vi "Motion UI.vi"() -> ()   [LabVIEW 2010]
uses:
  Motion_Gantry Position.ctl
  Motion_Coils Typedef.ctl
  Motion_Registers Typedef.ctl
  <vilib>/NI Modbus.llb/MB Ethernet Master Query Write Multiple Registers (poly).vi
panel:
  in  "Write Home data\n(All Axis)":bool
  in  "X Home Data":T1={"Approach Velocity (In/Sec)"=1.0, "Creep Velocity (In/Sec)"=0.5, "Offset (In)"=-0.0625, "OffsetVelocity (In/Sec)"=0.5, "AccDec\n(In/Sec/Sec)"=1.0, "Position (In)"=22.525} {"Position (In)" format="%.3f"; "AccDec\n(In/Sec/Sec)" min=0.01 max=20.0 format="%.2f"; "OffsetVelocity (In/Sec)" min=0.01 max=2.0 format="%.2f"; "Offset (In)" min=-1.0 max=1.0 format="%.3f"; "Creep Velocity (In/Sec)" min=0.5 max=1.0 format="%.2f"; "Approach Velocity (In/Sec)" min=0.01 max=2.0 format="%.2f"}
  in  "Y Home Data":T2={"Approach Velocity\n(In/Sec)"=1.0, "Creep Velocity\n(In/Sec)"=0.5, "Offset (In)"=-0.0625, "OffsetVelocity\n(In/Sec)"=0.5, "AccDec\n(In/Sec/Sec)"=1.0, "Position (In)"=5.9} {"Position (In)" format="%.3f"; "AccDec\n(In/Sec/Sec)" min=0.01 max=20.0 format="%.2f"; "OffsetVelocity\n(In/Sec)" min=0.01 max=2.0 format="%.2f"; "Offset (In)" min=-1.0 max=1.0 format="%.3f"; "Creep Velocity\n(In/Sec)" min=0.5 max=1.0 format="%.2f"; "Approach Velocity\n(In/Sec)" min=0.01 max=2.0 format="%.2f"}
  in  "Z Home Data":T2={"Approach Velocity\n(In/Sec)"=1.0, "Creep Velocity\n(In/Sec)"=0.5, "Offset (In)"=-0.0625, "OffsetVelocity\n(In/Sec)"=0.5, "AccDec\n(In/Sec/Sec)"=1.0, "Position (In)"=5.75} {"Position (In)" format="%.3f"; "AccDec\n(In/Sec/Sec)" min=0.01 max=20.0 format="%.2f"; "OffsetVelocity\n(In/Sec)" min=0.01 max=2.0 format="%.2f"; "Offset (In)" min=-1.0 format="%.3f"; "Creep Velocity\n(In/Sec)" min=0.5 max=1.0 format="%.2f"; "Approach Velocity\n(In/Sec)" min=0.01 max=2.0 format="%.2f"}
  in  "Loader Home Data":T2={"Approach Velocity\n(In/Sec)"=1.0, "Creep Velocity\n(In/Sec)"=0.5, "Offset (In)"=0.0625, "OffsetVelocity\n(In/Sec)"=0.5, "AccDec\n(In/Sec/Sec)"=1.0, "Position (In)"=0.0} {"Position (In)" min=0.0 max=1.0 format="%.3f"; "AccDec\n(In/Sec/Sec)" min=0.01 max=20.0 format="%.2f"; "OffsetVelocity\n(In/Sec)" min=0.01 max=2.0 format="%.2f"; "Offset (In)" min=-1.0 max=1.0 format="%.3f"; "Creep Velocity\n(In/Sec)" min=0.5 max=1.0 format="%.2f"; "Approach Velocity\n(In/Sec)" min=0.01 max=2.0 format="%.2f"}
  out "Errors":cluster{"Error ID":u16, "Error String":string}[](array[cluster])
  in  "General Alarm Clear":bool
  out "Loader Discretes":T3
  out "Gantry Discretes":T4
  out "Gantry Position":T5
  out "error out":errorcluster
  in  "stop":bool
  in  "address:port":string="192.168.0.3:502"
  in  "Gantry Move Data":T6={"Gantry Accel/Decel"=5.0, "Gantry Velocity"=5.0, "X-Position"=0.3, "Y-Position"=0.0, "Z-Position"=-0.5} {"Z-Position" format="%_7g"; "Y-Position" format="%_7g"; "X-Position" format="%_7g"; "Gantry Velocity" format="%_7g"; "Gantry Accel/Decel" format="%_7g"}
  out "Loader Actual Position":dbl format="%.3f"
  in  "Loader Stop":bool
  in  "Loader Goto Load":bool
  in  "Loader Goto Connect":bool
  in  "Loader Enable":bool
  in  "Loader Home":bool
  in  "Gantry Goto":bool
  in  "Gantry Home":bool
  in  "Gantry Enable":bool
  # "Loader Control"
  # "Gantry Control"
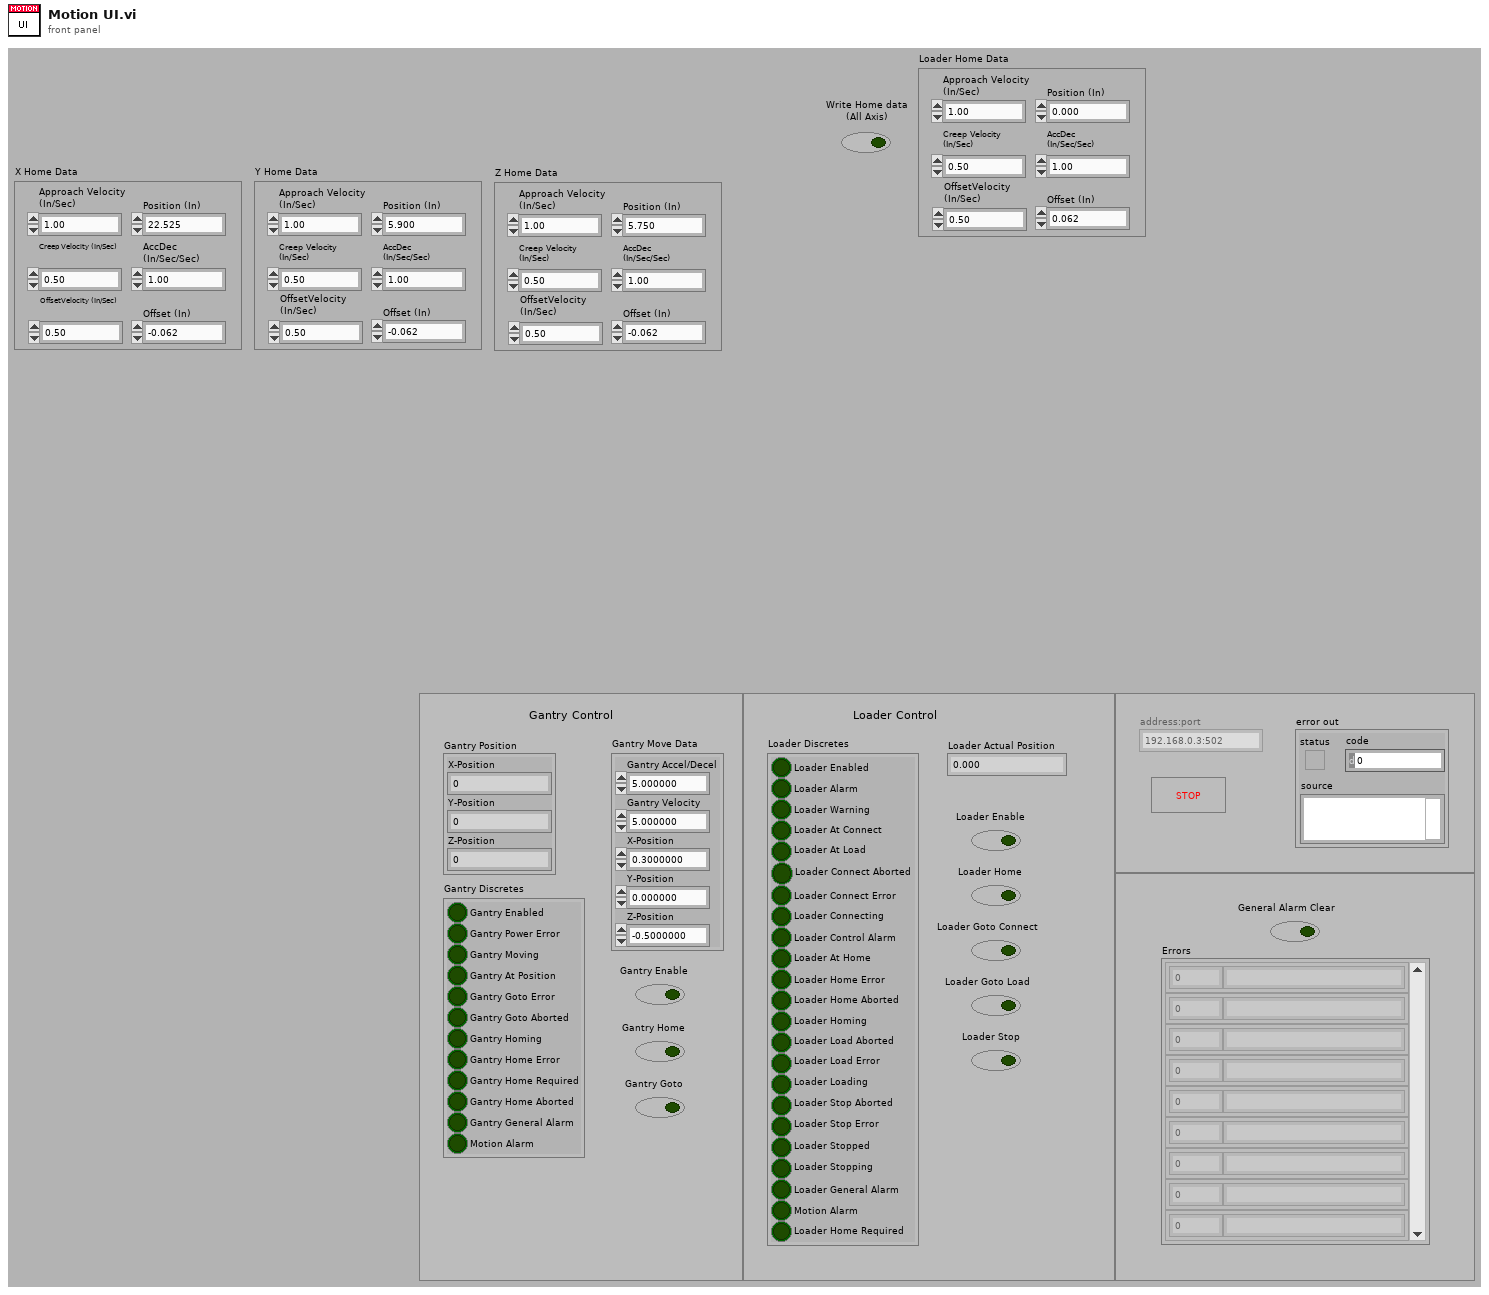
[diagram p1: front panel]
types:
  T1 = cluster{"Approach Velocity (In/Sec)":dbl, "Creep Velocity (In/Sec)":dbl, "Offset (In)":dbl, "OffsetVelocity (In/Sec)":dbl, "AccDec\n(In/Sec/Sec)":dbl, "Position (In)":dbl}
  T2 = cluster{"Approach Velocity\n(In/Sec)":dbl, "Creep Velocity\n(In/Sec)":dbl, "Offset (In)":dbl, "OffsetVelocity\n(In/Sec)":dbl, "AccDec\n(In/Sec/Sec)":dbl, "Position (In)":dbl}
  T3 = cluster{"Loader Enabled":bool, "Loader Alarm ":bool, "Loader Warning":bool, "Loader At Connect":bool, "Loader At Load":bool, "Loader Connect Aborted":bool, "Loader Connect Error":bool, "Loader Connecting":bool, "Loader Control Alarm":bool, "Loader At Home":bool, "Loader Home Error":bool, "Loader Home Aborted":bool, "Loader Homing":bool, "Loader Load Aborted":bool, "Loader Load Error":bool, "Loader Loading":bool, "Loader Stop Aborted":bool, "Loader Stop Error":bool, "Loader Stopped":bool, "Loader Stopping":bool, "Loader General Alarm":bool, "Motion Alarm":bool, "Loader Home Required":bool}
  T4 = cluster{"Gantry Enabled":bool, "Gantry Power Error":bool, "Gantry Moving":bool, "Gantry At Position":bool, "Gantry Goto Error":bool, "Gantry Goto Aborted":bool, "Gantry Homing":bool, "Gantry Home Error":bool, "Gantry Home Required":bool, "Gantry Home Aborted":bool, "Gantry General Alarm":bool, "Motion Alarm":bool}
  T5 = cluster{"X-Position":dbl, "Y-Position":dbl, "Z-Position":dbl}
  T6 = typedef "Motion_Gantry Position.ctl" = cluster{"Gantry Accel/Decel":dbl, "Gantry Velocity":dbl, "X-Position":dbl, "Y-Position":dbl, "Z-Position":dbl}
  T7 = typedef "Motion_Coils Typedef.ctl" = u16
  T8 = typedef "Motion_Registers Typedef.ctl" = u16
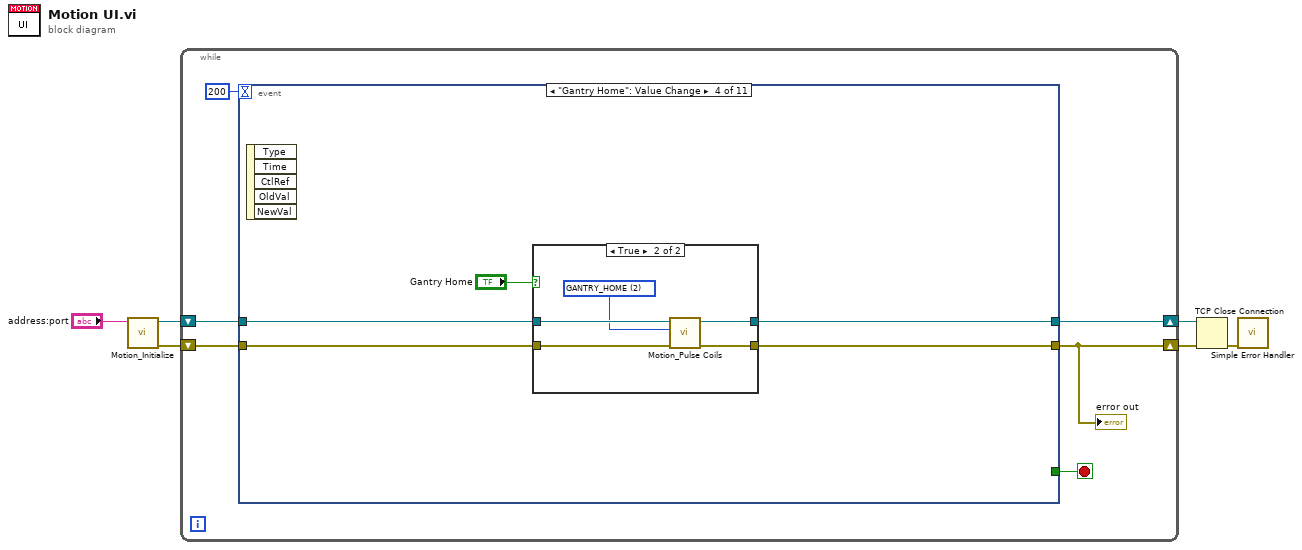
[diagram p0: block diagram]
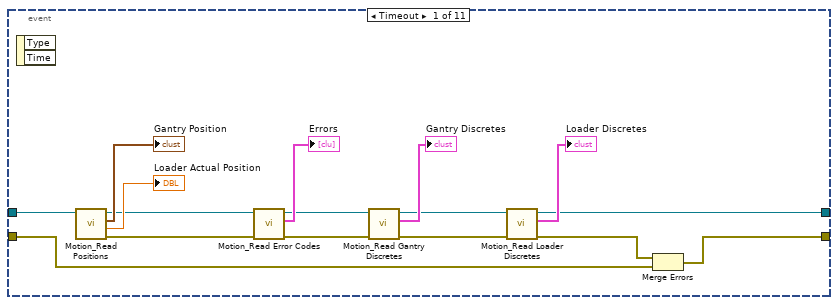
[diagram p2: hidden frame]
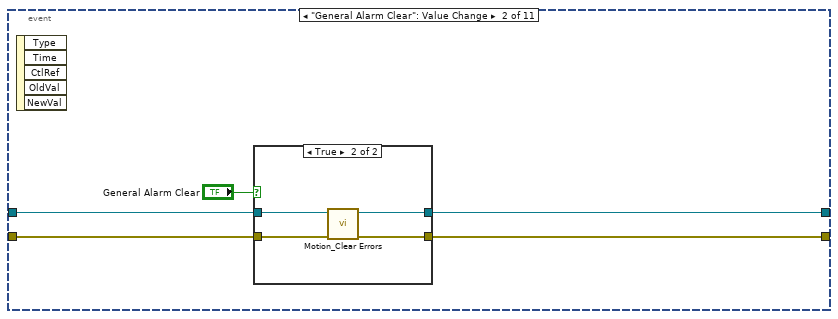
[diagram p3: hidden frame]
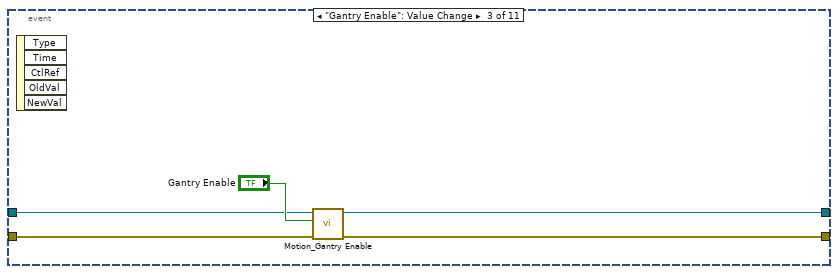
[diagram p5: hidden frame]
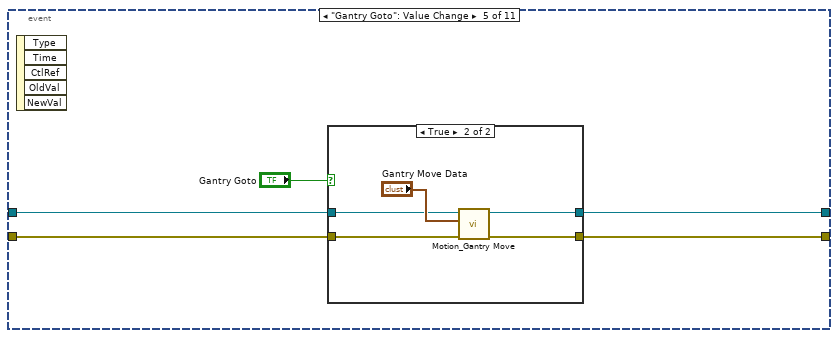
[diagram p7: hidden frame]
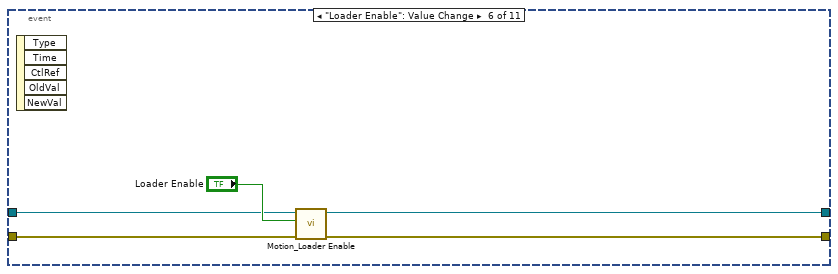
[diagram p9: hidden frame]
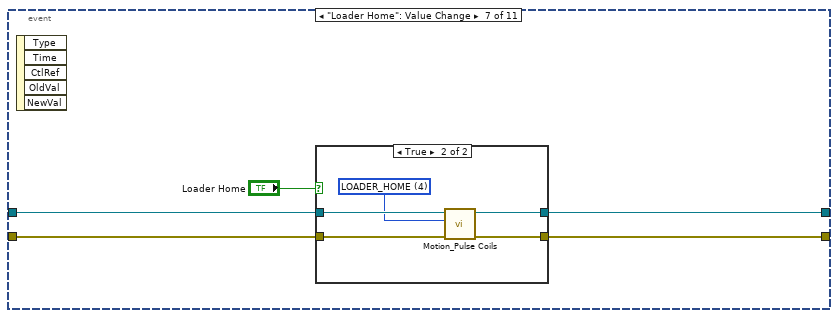
[diagram p10: hidden frame]
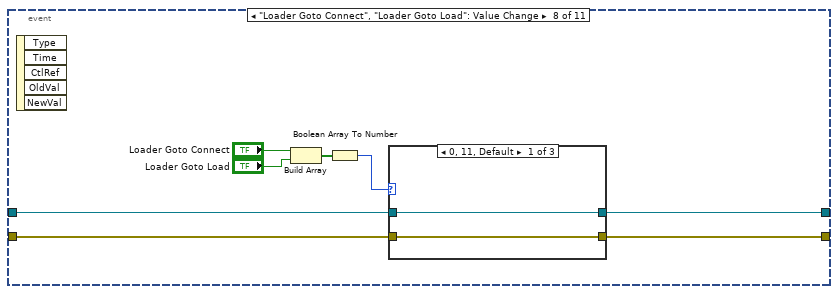
[diagram p12: hidden frame]
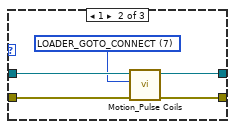
[diagram p13: hidden frame]
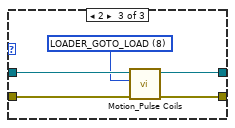
[diagram p14: hidden frame]
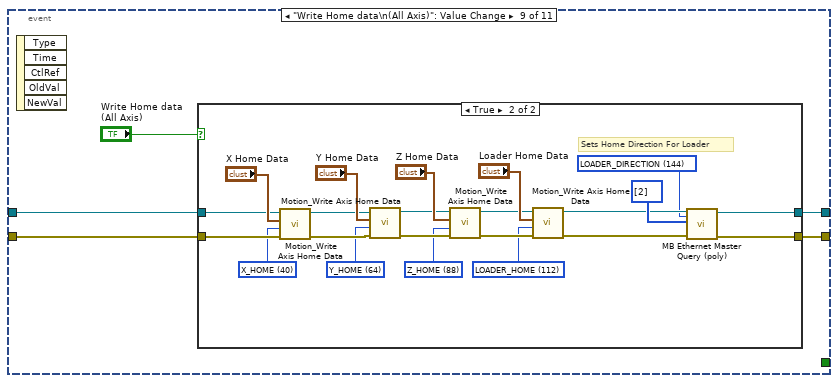
[diagram p15: hidden frame]
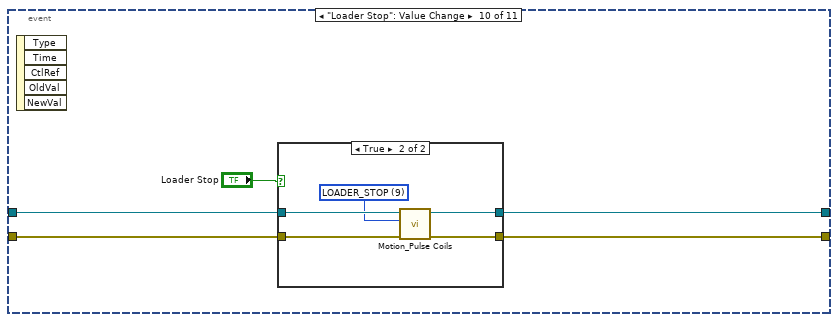
[diagram p17: hidden frame]
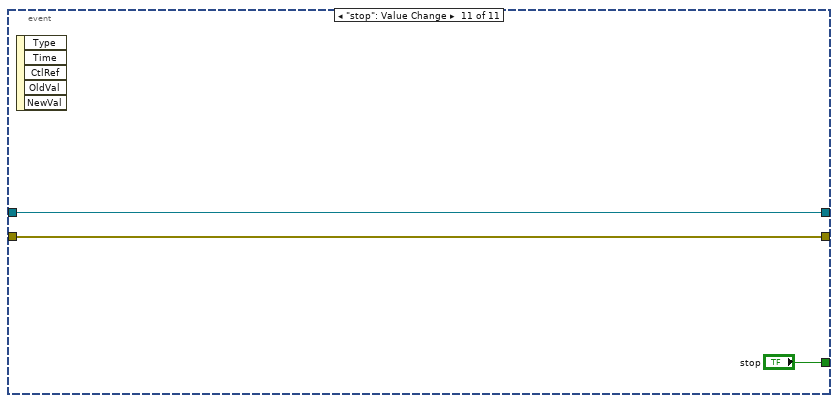
[diagram p19: hidden frame]
diagram:
  n1 = call "Motion_Initialize.vi"("TCP address:port (192.168.0.3:502)"="address:port") -> ("error out"=w4:errorcluster, "connection ID"=w3:refnum<k5>)  [unwired: 9 in]
  n2 = while {
    shift-right: [w9] -> w1
    shift-left: w3 -> [w10]
    shift-right: [w8] -> w2
    shift-left: w4 -> [w11]
    stop <- w12 stop-if-true
    n3 = event shown="[3] \"Gantry Home\": Value Change" {
      selector: _ -> [_ _ _ _ _ _ _ _ _ _ _]
      dyn-events: _ -> [_ _ _ _ _ _ _ _ _ _ _]
      timeout: 200 -> [_ _ _ _ _ _ _ _ _ _ _]
      tunnel: [_ _ _ _ _ _ _ _ _ _ "stop"] -> w12
      tunnel: w11 -> [w15 w32 w43 w47 w60 w73 w78 w89 w109 w139 w149]
      tunnel: [w13 w31 w41 w46 w59 w72 w77 w88 w106 w136 w149] -> w8
      tunnel: w10 -> [w17 w30 w42 w49 w61 w69 w76 w87 w108 w138 w147]
      tunnel: [w16 w29 w40 w48 w58 w71 w75 w86 w107 w137 w147] -> w9
      event Timeout {
        n4 = event-data() -> ()  [unwired: 1 in, 2 out]
        n5 = call "Motion_Read Positions.vi"("TCP Connection Refnum in"=w17) -> ("error out"=w19:errorcluster, "Loader Position"=→"Loader Actual Position":dbl, "Gantry Position"=→"Gantry Position":T5, "TCP Connection Refnum (dup)"=w18:refnum<k5>)  [unwired: 5 in, 2 out]
        n6 = call "Motion_Read Error Codes.vi"("error in (no error)"=w19, "TCP Connection Refnum in"=w18) -> ("error out"=w23:errorcluster, "Errors"=→"Errors":cluster{"Error ID":u16, "Error String":string}[], "TCP Connection Refnum (dup)"=w22:refnum<k5>)  [unwired: 6 in, 1 out]
        n7 = call "Motion_Read Gantry Discretes.vi"("error in (no error)"=w23, "TCP Connection Refnum in"=w22) -> ("error out"=w25:errorcluster, "Gantry Discretes"=→"Gantry Discretes":T4, "TCP Connection Refnum (dup)"=w24:refnum<k5>)  [unwired: 7 in]
        n8 = call "Motion_Read Loader Discretes.vi"("error in (no error)"=w25, "TCP Connection Refnum in"=w24) -> ("error out"=w14:errorcluster, "Loader Discretes"=→"Loader Discretes":T3, "TCP Connection Refnum (dup)"=w16:refnum<k5>)  [unwired: 7 in]
        n9 = Merge Errors(w14, w15) -> (w13:errorcluster)
      }
      event "General Alarm Clear": Value Change {
        n10 = event-data() -> ()  [unwired: 1 in, 5 out]
        n11 = case shown="True" "General Alarm Clear" {
          tunnel: w32 -> [w34 w39]
          tunnel: [w34 w38] -> w31
          tunnel: w30 -> [w35 w37]
          tunnel: [w35 w36] -> w29
          frame False {
          }
          frame True {
            n12 = call "Motion_Clear Errors.vi"("error in (no error)"=w39, "TCP Connection Refnum in"=w37) -> ("error out"=w38:errorcluster, "TCP Connection Refnum (dup)"=w36:refnum<k5>)  [unwired: 8 in]
          }
        }
      }
      event "Gantry Enable": Value Change {
        n13 = event-data() -> ()  [unwired: 1 in, 5 out]
        n14 = call "Motion_Gantry Enable.vi"("error in (no error)"=w43, "Enable? (T)"="Gantry Enable", "TCP Connection Refnum in"=w42) -> ("error out"=w41:errorcluster, "TCP Connection Refnum (dup)"=w40:refnum<k5>)  [unwired: 7 in]
      }
      event "Gantry Home": Value Change {
        n15 = event-data() -> ()  [unwired: 1 in, 5 out]
        n16 = case shown="True" "Gantry Home" {
          tunnel: w49 -> [w51 w56]
          tunnel: [w51 w55] -> w48
          tunnel: w47 -> [w50 w52]
          tunnel: [w50 w54] -> w46
          frame False {
          }
          frame True {
            w53 = T7 2 items=["GANTRY_ALARM_CLEAR", "GANTRY_ENABLE", "GANTRY_HOME", "GANTRY_GOTO", "LOADER_HOME", "LOADER_ALARM_CLEAR", "LOADER_ENABLE", "LOADER_GOTO_CONNECT", "LOADER_GOTO_LOAD", "LOADER_STOP"] ("Coils")
            n17 = call "Motion_Pulse Coils.vi"("error in"=w52, "Pulse Coil"=w53, "TCP refnum"=w56) -> ("error out"=w54:errorcluster, "TCP refnum dup"=w55:refnum<k5>)  [unwired: 7 in]
          }
        }
      }
      event "Gantry Goto": Value Change {
        n18 = event-data() -> ()  [unwired: 1 in, 5 out]
        n19 = case shown="True" "Gantry Goto" {
          tunnel: w61 -> [w63 w67]
          tunnel: w60 -> [w62 w66]
          tunnel: [w62 w65] -> w59
          tunnel: [w63 w64] -> w58
          frame False {
          }
          frame True {
            n20 = call "Motion_Gantry Move.vi"("error in (no error)"=w66, "Gantry Move Data"="Gantry Move Data", "TCP Connection Refnum in"=w67) -> ("error out"=w65:errorcluster, "TCP Connection Refnum (dup)"=w64:refnum<k5>)  [unwired: 7 in]
          }
        }
      }
      event "Loader Enable": Value Change {
        n21 = event-data() -> ()  [unwired: 1 in, 5 out]
        n22 = call "Motion_Loader Enable.vi"("error in (no error)"=w73, "Enable? (T)"="Loader Enable", "TCP Connection Refnum in"=w69) -> ("error out"=w72:errorcluster, "TCP Connection Refnum (dup)"=w71:refnum<k5>)  [unwired: 7 in]
      }
      event "Loader Home": Value Change {
        n23 = event-data() -> ()  [unwired: 1 in, 5 out]
        n24 = case shown="True" "Loader Home" {
          tunnel: w78 -> [w79 w85]
          tunnel: [w79 w84] -> w77
          tunnel: w76 -> [w80 w83]
          tunnel: [w80 w82] -> w75
          frame False {
          }
          frame True {
            w81 = T7 4 items=["GANTRY_ALARM_CLEAR", "GANTRY_ENABLE", "GANTRY_HOME", "GANTRY_GOTO", "LOADER_HOME", "LOADER_ALARM_CLEAR", "LOADER_ENABLE", "LOADER_GOTO_CONNECT", "LOADER_GOTO_LOAD", "LOADER_STOP"] ("Coils")
            n25 = call "Motion_Pulse Coils.vi"("error in"=w85, "Pulse Coil"=w81, "TCP refnum"=w83) -> ("error out"=w84:errorcluster, "TCP refnum dup"=w82:refnum<k5>)  [unwired: 7 in]
          }
        }
      }
      event "Loader Goto Connect", "Loader Goto Load": Value Change {
        n26 = event-data() -> ()  [unwired: 1 in, 5 out]
        n27 = Build Array("Loader Goto Connect", "Loader Goto Load") -> (w91:bool[])
        n28 = Boolean Array To Number(Boolean array=w91) -> (number=w90:u32)
        n29 = case shown="0, 11, Default" w90 {
          tunnel: w89 -> [w95 w100 w105]
          tunnel: [w95 w99 w104] -> w88
          tunnel: w87 -> [w94 w98 w103]
          tunnel: [w94 w97 w102] -> w86
          frame 0, 3, Default {
          }
          frame 1 {
            w96 = T7 7 items=["GANTRY_ALARM_CLEAR", "GANTRY_ENABLE", "GANTRY_HOME", "GANTRY_GOTO", "LOADER_HOME", "LOADER_ALARM_CLEAR", "LOADER_ENABLE", "LOADER_GOTO_CONNECT", "LOADER_GOTO_LOAD", "LOADER_STOP"] ("Pulse Coil")
            n30 = call "Motion_Pulse Coils.vi"("error in"=w100, "Pulse Coil"=w96, "TCP refnum"=w98) -> ("error out"=w99:errorcluster, "TCP refnum dup"=w97:refnum<k5>)  [unwired: 7 in]
          }
          frame 2 {
            w101 = T7 8 items=["GANTRY_ALARM_CLEAR", "GANTRY_ENABLE", "GANTRY_HOME", "GANTRY_GOTO", "LOADER_HOME", "LOADER_ALARM_CLEAR", "LOADER_ENABLE", "LOADER_GOTO_CONNECT", "LOADER_GOTO_LOAD", "LOADER_STOP"] ("Pulse Coil")
            n31 = call "Motion_Pulse Coils.vi"("error in"=w105, "Pulse Coil"=w101, "TCP refnum"=w103) -> ("error out"=w104:errorcluster, "TCP refnum dup"=w102:refnum<k5>)  [unwired: 7 in]
          }
        }
      }
      event "Write Home data\n(All Axis)": Value Change {
        n32 = event-data() -> ()  [unwired: 1 in, 5 out]
        n33 = case shown="True" "Write Home data\n(All Axis)" {
          tunnel: [w111 w121] -> w106
          tunnel: [w112 w120] -> w107
          tunnel: w109 -> [w111 w119]
          tunnel: w108 -> [w112 w118]
          frame False {
          }
          frame True {
            w116 = T8 144 items=["GANTRY_MOTION"=20, "X_HOME"=40, "Y_HOME"=64, "Z_HOME"=88, "LOADER_HOME"=112, "LOADER_DIRECTION"=144] ("Registers")
            w115 = T8 112 items=["GANTRY_MOTION"=20, "X_HOME"=40, "Y_HOME"=64, "Z_HOME"=88, "LOADER_HOME"=112, "LOADER_DIRECTION"=144] ("Registers")
            w114 = T8 88 items=["GANTRY_MOTION"=20, "X_HOME"=40, "Y_HOME"=64, "Z_HOME"=88, "LOADER_HOME"=112, "LOADER_DIRECTION"=144] ("Registers")
            w113 = T8 64 items=["GANTRY_MOTION"=20, "X_HOME"=40, "Y_HOME"=64, "Z_HOME"=88, "LOADER_HOME"=112, "LOADER_DIRECTION"=144] ("Registers")
            w117 = T8 40 items=["GANTRY_MOTION"=20, "X_HOME"=40, "Y_HOME"=64, "Z_HOME"=88, "LOADER_HOME"=112, "LOADER_DIRECTION"=144] ("Registers")
            # "Sets Home Direction For Loader"
            n34 = call "Motion_Write Axis Home Data.vi"("error in"=w119, "Register"=w117, "Home Data"="X Home Data", "TCP Connection Refnum in"=w118) -> ("error out"=w125:errorcluster, "TCP Connection Refnum (dup)"=w129:refnum<k5>)  [unwired: 6 in]
            n35 = call "Motion_Write Axis Home Data.vi"("error in"=w125, "Register"=w113, "Home Data"="Y Home Data", "TCP Connection Refnum in"=w129) -> ("error out"=w124:errorcluster, "TCP Connection Refnum (dup)"=w128:refnum<k5>)  [unwired: 6 in]
            n36 = call "Motion_Write Axis Home Data.vi"("error in"=w124, "Register"=w114, "Home Data"="Z Home Data", "TCP Connection Refnum in"=w128) -> ("error out"=w123:errorcluster, "TCP Connection Refnum (dup)"=w127:refnum<k5>)  [unwired: 6 in]
            n37 = call "Motion_Write Axis Home Data.vi"("error in"=w123, "Register"=w115, "Home Data"="Loader Home Data", "TCP Connection Refnum in"=w127) -> ("error out"=w122:errorcluster, "TCP Connection Refnum (dup)"=w126:refnum<k5>)  [unwired: 6 in]
            n38 = call-poly <vilib>:"MB Ethernet Master Query (poly).vi"("TCP Connection Refnum in"=w126, "Starting Address"=w116, "Registers"=u16[] [2], "error in"=w122) -> ("TCP Connection Refnum (dup)"=w120:refnum<k5>, "error out"=w121:errorcluster)  [unwired: 13 in, 1 out]
          }
        }
      }
      event "Loader Stop": Value Change {
        n39 = event-data() -> ()  [unwired: 1 in, 5 out]
        n40 = case shown="True" "Loader Stop" {
          tunnel: w139 -> [w140 w146]
          tunnel: w138 -> [w141 w145]
          tunnel: [w141 w144] -> w137
          tunnel: [w140 w143] -> w136
          frame False {
          }
          frame True {
            w142 = T7 9 items=["GANTRY_ALARM_CLEAR", "GANTRY_ENABLE", "GANTRY_HOME", "GANTRY_GOTO", "LOADER_HOME", "LOADER_ALARM_CLEAR", "LOADER_ENABLE", "LOADER_GOTO_CONNECT", "LOADER_GOTO_LOAD", "LOADER_STOP"] ("Coils")
            n41 = call "Motion_Pulse Coils.vi"("error in"=w146, "Pulse Coil"=w142, "TCP refnum"=w145) -> ("error out"=w143:errorcluster, "TCP refnum dup"=w144:refnum<k5>)  [unwired: 7 in]
          }
        }
      }
      event "stop": Value Change {
        n42 = event-data() -> ()  [unwired: 1 in, 5 out]
      }
    }
    "error out" <- w8
  }
  n43 = TCP Close Connection(connection ID=w1, error in (no error)=w2) -> (error out=w6:errorcluster)  [unwired: 1 in, 1 out]
  n44 = call <vilib>:"Simple Error Handler.vi"("error in (no error)"=w6) -> ()  [unwired: 4 in, 5 out]
